vi "RunTest.vi"(8 "error in (no error)":errorcluster, 11 "Test In":refnum<class "Test.lvclass">) -> (0 "error out":errorcluster, 3 "Test Out":refnum<class "Test.lvclass">)   [LabVIEW 2017, in "Test.lvclass"]
doc: "Override to run the test and assert its state."
uses:
  Test.lvclass
  <vilib>/ErrorRing/Error Ring.xnode
  <vilib>/Utility/error.llb/Error Cluster From Error Code.vi
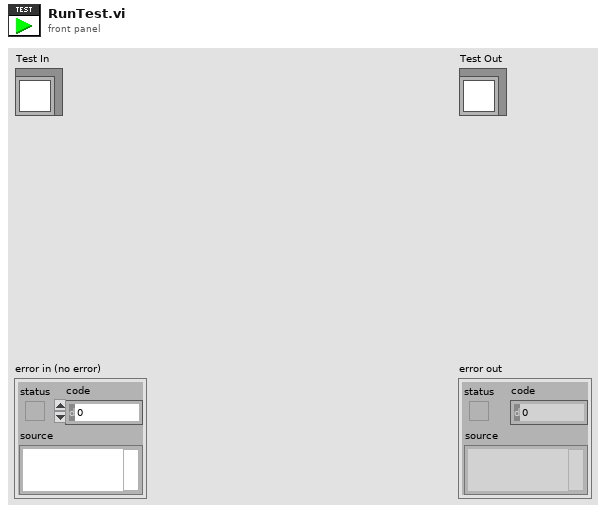
[diagram p1: front panel]
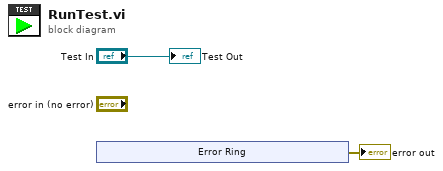
[diagram p0: block diagram]
diagram:
  n1 = xnode "Error Ring"() -> ("error out"=→"error out":errorcluster)
  "Test Out" <- "Test In"
